vi "Is value NaN or Inf.vi"(3 "Value":dbl) -> (1 "NaN or Inf":bool)   [LabVIEW 2017]
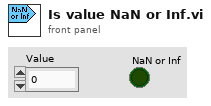
[diagram p1: front panel]
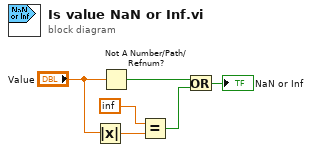
[diagram p0: block diagram]
diagram:
  n1 = Absolute Value(x="Value") -> (abs(x)=w4:dbl)
  n2 = Not A Number/Path/Refnum?(number/path/refnum="Value") -> (NaN/Path/Refnum?=w5:bool)
  n3 = Equal?(x=inf, y=w4) -> (x = y?=w1:bool)
  n4 = Or(x=w5, y=w1) -> (x .or. y?=→"NaN or Inf":bool)
